vi "Build.vi"(9 "XYZTheta":dbl[](array[numeric]), 10 "Pattern Coordinates":dbl[][](array[numeric]), 11 "C4 Dispense in":refnum<class "Iterative Dispense.lvclass">) -> (1 "Starting Coordinates":dbl[](array[numeric]), 3 "C4 Dispense out":refnum<class "Iterative Dispense.lvclass">)   [LabVIEW 2016, in "Iterative Dispense.lvclass"]
uses:
  Iterative Dispense.lvclass
  Iterative Dispense.lvclass/Iterative Dispense.ctl
  <vilib>/Analysis/coordinate.llb/2D Cartesian Coordinate Rotation (Array).vi
  <vilib>/Analysis/NI_AALPro.lvlib
panel:
  out "array w/ subset deleted":dbl[][][](array[numeric])
  out "deleted portion":dbl[][](array[numeric])
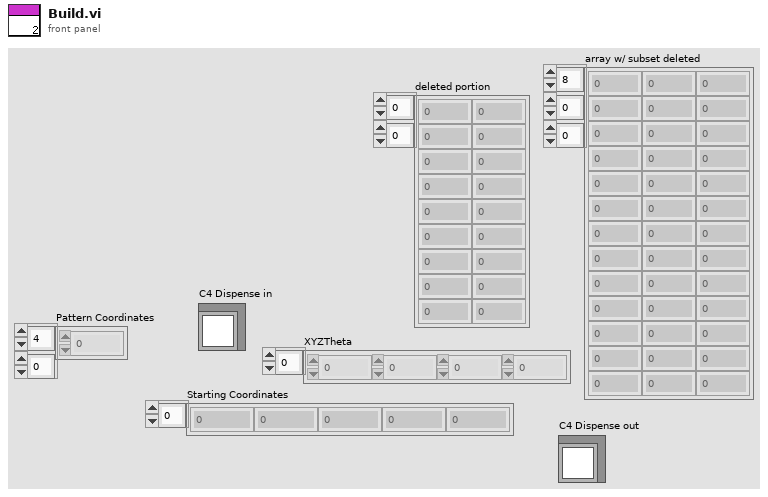
[diagram p1: front panel]
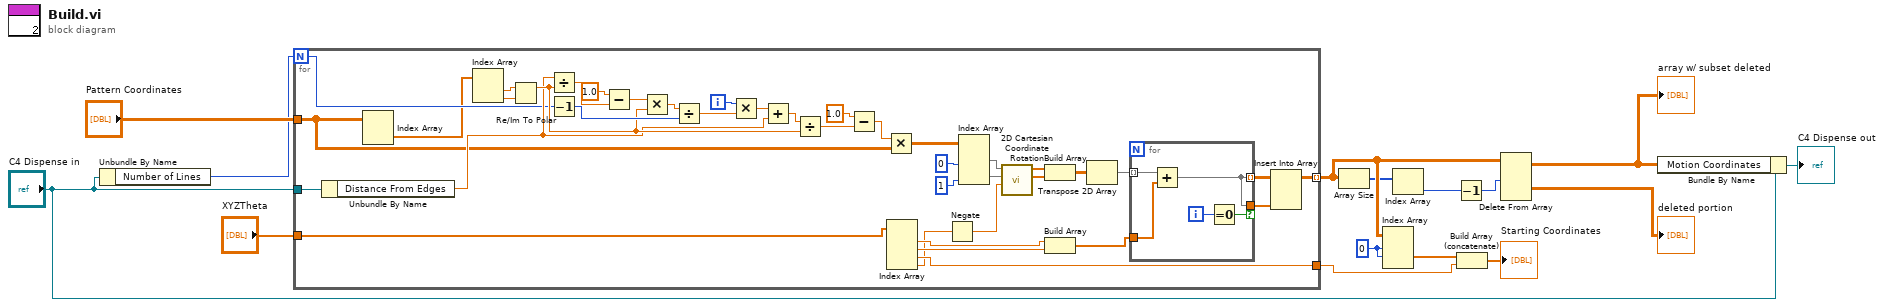
[diagram p0: block diagram]
diagram:
  w15 = 0 ("disabled index (page)")
  n1 = Unbundle By Name("C4 Dispense in") -> ("Number of Lines"=w9:i32)
  n2 = for {
    N: w9 -> [w30]
    tunnel: [w24] -> w5 mode=indexing
    tunnel: "XYZTheta" -> [w32]
    tunnel: "C4 Dispense in" -> [w36]
    tunnel: "Pattern Coordinates" -> [w23]
    tunnel: [w29] -> w12
    i -> [w49]
    n3 = Unbundle By Name(w36) -> ("Distance From Edges"=w35:dbl)
    n4 = Index Array(array=w23) -> (element=w22:dbl[])  [unwired: 2 in]
    n5 = Index Array(array=w22) -> (element #1=w21:dbl, element #2=w20:dbl)  [unwired: 2 in]
    n6 = Re/Im To Polar(2:w20, 3:w21) -> (1:w37:dbl)  [unwired: 1 out]
    n7 = Divide(x=w35, y=w37) -> (x/y=w43:dbl)
    n8 = Decrement(x=w30) -> (x-1=w39:i32)
    n9 = Subtract(x=1.0, y=w43) -> (x-y=w41:dbl)
    n10 = Multiply(x=w41, y=w37) -> (x*y=w40:dbl)
    n11 = Divide(x=w40, y=w39) -> (x/y=w38:dbl)
    n12 = Multiply(x=w49, y=w38) -> (x*y=w54:dbl)
    n13 = Add(x=w54, y=w35) -> (x+y=w53:dbl)
    n14 = Divide(x=w53, y=w37) -> (x/y=w52:dbl)
    n15 = Subtract(x=1.0, y=w52) -> (x-y=w44:dbl)
    n16 = Multiply(x=w44, y=w23) -> (x*y=w50:dbl[][])
    n17 = Index Array(array=w32) -> (element #1=w34:dbl, element #2=w33:dbl, element #3=w29:dbl, element #4=w17:dbl)  [unwired: 4 in]
    n18 = Negate(x=w17) -> (-x=w16:dbl)
    n19 = Index Array(array=w50, index (col) #1=0 ("disabled index (col)"), index (col) #2=1 ("index (col)")) -> (element #1=w28:dbl[], element #2=w27:dbl[])  [unwired: 2 in]
    n20 = call-poly <vilib>:"2D Cartesian Coordinate Rotation.vi"("theta"=w16, "Y"=w27, "X"=w28) -> ("Y Out"=w48:dbl[], "X Out"=w47:dbl[])  [unwired: 6 in, 1 out]
    n21 = Build Array(w47, w48) -> (w19:dbl[][])
    n22 = Build Array(w34, w33) -> (w31:dbl[])
    n23 = Transpose 2D Array(2D array=w19) -> (transposed array=w18:dbl[][])
    n24 = for {
      tunnel: w31 -> [w59]
      tunnel: w18 -> [w58] mode=indexing
      tunnel: [w55] -> w26 mode=indexing
      tunnel: [w55] -> w25 if=w56
      i -> [w57]
      n25 = Add(x=w58, y=w59) -> (x+y=w55:dbl[])
      n26 = Equal To 0?(x=w57) -> (x = 0?=w56:bool)
    }
    n27 = Insert Into Array(array=w26, new element=w25) -> (w24:dbl[][])  [unwired: 2 in]
  }
  n28 = Array Size(array=w5) -> (size(s)=w4:i32[])
  n29 = Index Array "Index Array"(array=w5, index (dim 0)=w15, index (dim 1)=w15) -> (element=w13:dbl[])  [unwired: 1 in]
  n30 = Index Array(array=w4) -> (element=w2:i32)  [unwired: 1 in]
  n31 = Decrement(x=w2) -> (x-1=w1:i32)
  n32 = Build Array (concatenate)(w13, w12) -> (→"Starting Coordinates":dbl[])
  n33 = Delete From Array "Delete From Array"(array=w5, index (dim 0)=w1) -> (deleted portion=→"deleted portion":dbl[][], array with subset deleted=w6:dbl[][][])  [unwired: 3 in]
  "array w/ subset deleted" <- w6
  n34 = Bundle By Name(cluster="C4 Dispense in", "Motion Coordinates"=w6) -> (→"C4 Dispense out":refnum<class "Iterative Dispense.lvclass">)
